vi "Main.vi"(11 "Module Admin":refnum<class "Delacor_lib_QMH_Module Admin.lvclass">) -> ()   [LabVIEW 2023, in "DeviceManager.lvlib"]
doc: "This template is based off of the Queued Message Handler design pattern and the Queued Message Handler project template that ships with LabVIEW.\n\nThe main difference is that the queue is private to this module and communication between modules is performed via Broadcast and Request events.\n\nRequest events are wrapped in public API methods and are handled in the Event Handling Loop (EHL) of this VI. Any module can register for Broadcast events sent by this module. The EHL generates messages based on user interface actions.\n\nThe Message Handling Loop (MHL) processes messages generated by the EHL, or by other messages. The messages are string values, so new messages can be added easily to the Message Cases case structure in the MHL. Each message cluster can also provide an optional value for Message Data, which is a variant that can be converted to whatever message-specific data is required.\n_____\nBased on DQMH Project Template 7.0.0.1280."
uses:
  DeviceManager.lvlib
  <vilib>/Delacor/Delacor QMH/Libraries/Module Admin_class/Delacor_lib_QMH_Module Admin.lvclass
  Module Data--cluster.ctl
  ICLcommuncationData.ctl
  Communicator/Communicator.lvclass
  OpenWebSocketCommunication (Reply Payload)--cluster.ctl
  SendJSONandAskForReply (Reply Payload)--cluster.ctl
  DiscoverDevices (Reply Payload)--cluster.ctl
  Mono/Monochromator.lvclass
  CCD/CCD.lvclass
  SCD/SCD.lvclass
  DevicesList (Reply Payload)--cluster.ctl
  <vilib>/Delacor/Delacor QMH/Libraries/Message Queue_class/Delacor_lib_QMH_Message Queue.lvclass/Delacor_lib_QMH_Message Queue.ctl
  Stop Argument--cluster.ctl
  <vilib>/Delacor/Delacor QMH/Libraries/Module Admin_class/Delacor_lib_QMH_Module Admin.lvclass/Delacor_lib_QMH_Module Admin.ctl
  <vilib>/Utility/miscctls.llb/LVPointTypeDef.ctl
  18cac8b0-4f25-4128-b3b0-f125cc614320.vi
  <vilib>/Delacor/Delacor QMH/Libraries/Message Queue_class/Delacor_lib_QMH_Enqueue Message (Single).vi
  <vilib>/Delacor/Delacor QMH/Libraries/Module Admin_class/Delacor_lib_QMH_Get External Launch.vi
  522d4d4e-e2b9-4a0b-813b-57f0bcdbaa64.vi
  <vilib>/GPower/Error/Library/ErrorType.vi
  <vilib>/GPower/Error/Library/SplitAppended.vi
  <vilib>/Utility/error.llb/Trim Whitespace.vi
  <vilib>/GPower/Error/Library/SubVIs/ExplanationToError.vi
  <vilib>/Utility/error.llb/Trim Whitespace One-Sided.vi
  <vilib>/dlg_ctls.llb/Space Constant.vi
  <vilib>/Utility/error.llb/Error Code Database.vi
  <vilib>/GPower/Error/Library/SubVIs/SetStatus.vi
  <vilib>/GPower/Error/Library/AppendErrors.vi
  <vilib>/GPower/Error/Library/Append/AppendSingle.vi
  <vilib>/Delacor/Delacor QMH/Libraries/Message Queue_class/Delacor_lib_QMH_Message Queue.lvclass
  <vilib>/JKI/JKI DotNet System Exec/dotnet_system_exec/dotnet_system_exec.lvclass
  <vilib>/GPower/Error/GPError.lvlib
panel:
  out "ICL output":string caption="StdErr"
  out "StdOut":string
  out "error out":errorcluster
  out "Status":string
  in  "Simulate MHL Error":bool
  in  "Simulate EHL Error":bool
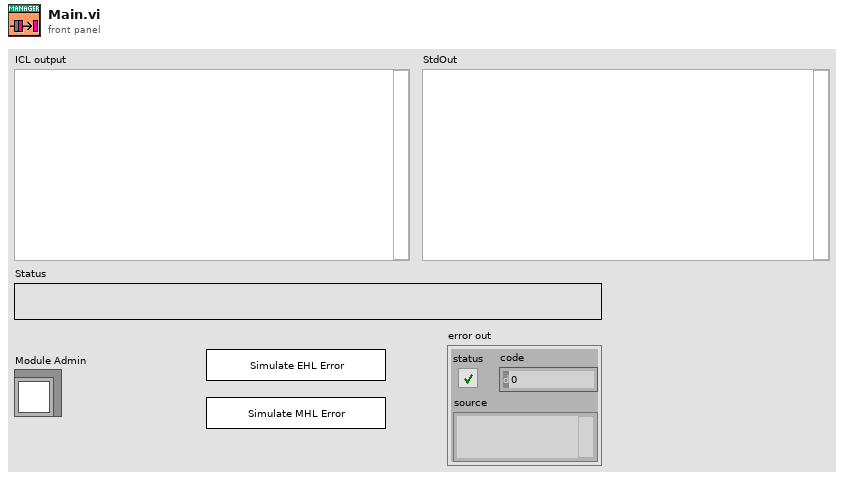
[diagram p1: front panel]
types:
  T1 = cluster{"stdout event":refnum<user-event>, "stderr event":refnum<user-event>, "process_exit event":refnum<user-event>}
  T2 = typedef "DeviceManager.lvlib/Request Events--cluster.ctl" = cluster{"Stop Module":refnum<user-event>, "Show Panel":refnum<user-event>, "Hide Panel":refnum<user-event>, "Get Module Execution Status":refnum<user-event>, "Show Diagram":refnum<user-event>, "StartICL":refnum<user-event>, "OpenWebSocketCommunication":refnum<user-event>, "Private":cluster{"ICLstartNotification":refnum<user-event>}, "ICLshutdown":refnum<user-event>, "SendJSONandAskForReply":refnum<user-event>, "DiscoverDevices":refnum<user-event>, "DevicesList":refnum<user-event>}
  T3 = typedef "DeviceManager.lvlib/ICLcommuncationData.ctl" = cluster{"Status":string, "ICL.exe started":bool, "Communicator":refnum<class "Communicator.lvclass">}
  T4 = typedef "DeviceManager.lvlib/Module Data--cluster.ctl" = cluster{"Status":string}
  T5 = typedef "DeviceManager.lvlib/OpenWebSocketCommunication (Reply Payload)--cluster.ctl" = cluster{"Return Headers":variant, "error":errorcluster}
  T6 = typedef "DeviceManager.lvlib/SendJSONandAskForReply (Reply Payload)--cluster.ctl" = cluster{"JSON reply":string, "error":errorcluster}
  T7 = typedef "DeviceManager.lvlib/DiscoverDevices (Reply Payload)--cluster.ctl" = cluster{"Monos":refnum<class "Monochromator.lvclass">[], "CCDs":refnum<class "CCD.lvclass">[], "SCDs":refnum<class "SCD.lvclass">[], "error":errorcluster}
  T8 = typedef "DeviceManager.lvlib/DevicesList (Reply Payload)--cluster.ctl" = cluster{"monochromator results":string, "CCD-results":string, "SCD-results":string, "error":errorcluster}
  T9 = enum32{"invalid lock state", "Not Locked", "Locked (No Password)", "Password-protected"}
  T10 = typedef "DeviceManager.lvlib/Stop Argument--cluster.ctl" = cluster{"Origin":string, "Exit via Stop Module Req?":bool, "Wait for Module to stop?":bool}
  T11 = typedef "LVPointTypeDef.ctl" = cluster{"Horizontal":i16, "Vertical":i16}
  T12 = enum32{"Invalid", "Standard", "Closed", "Hidden", "Minimized", "Maximized"}
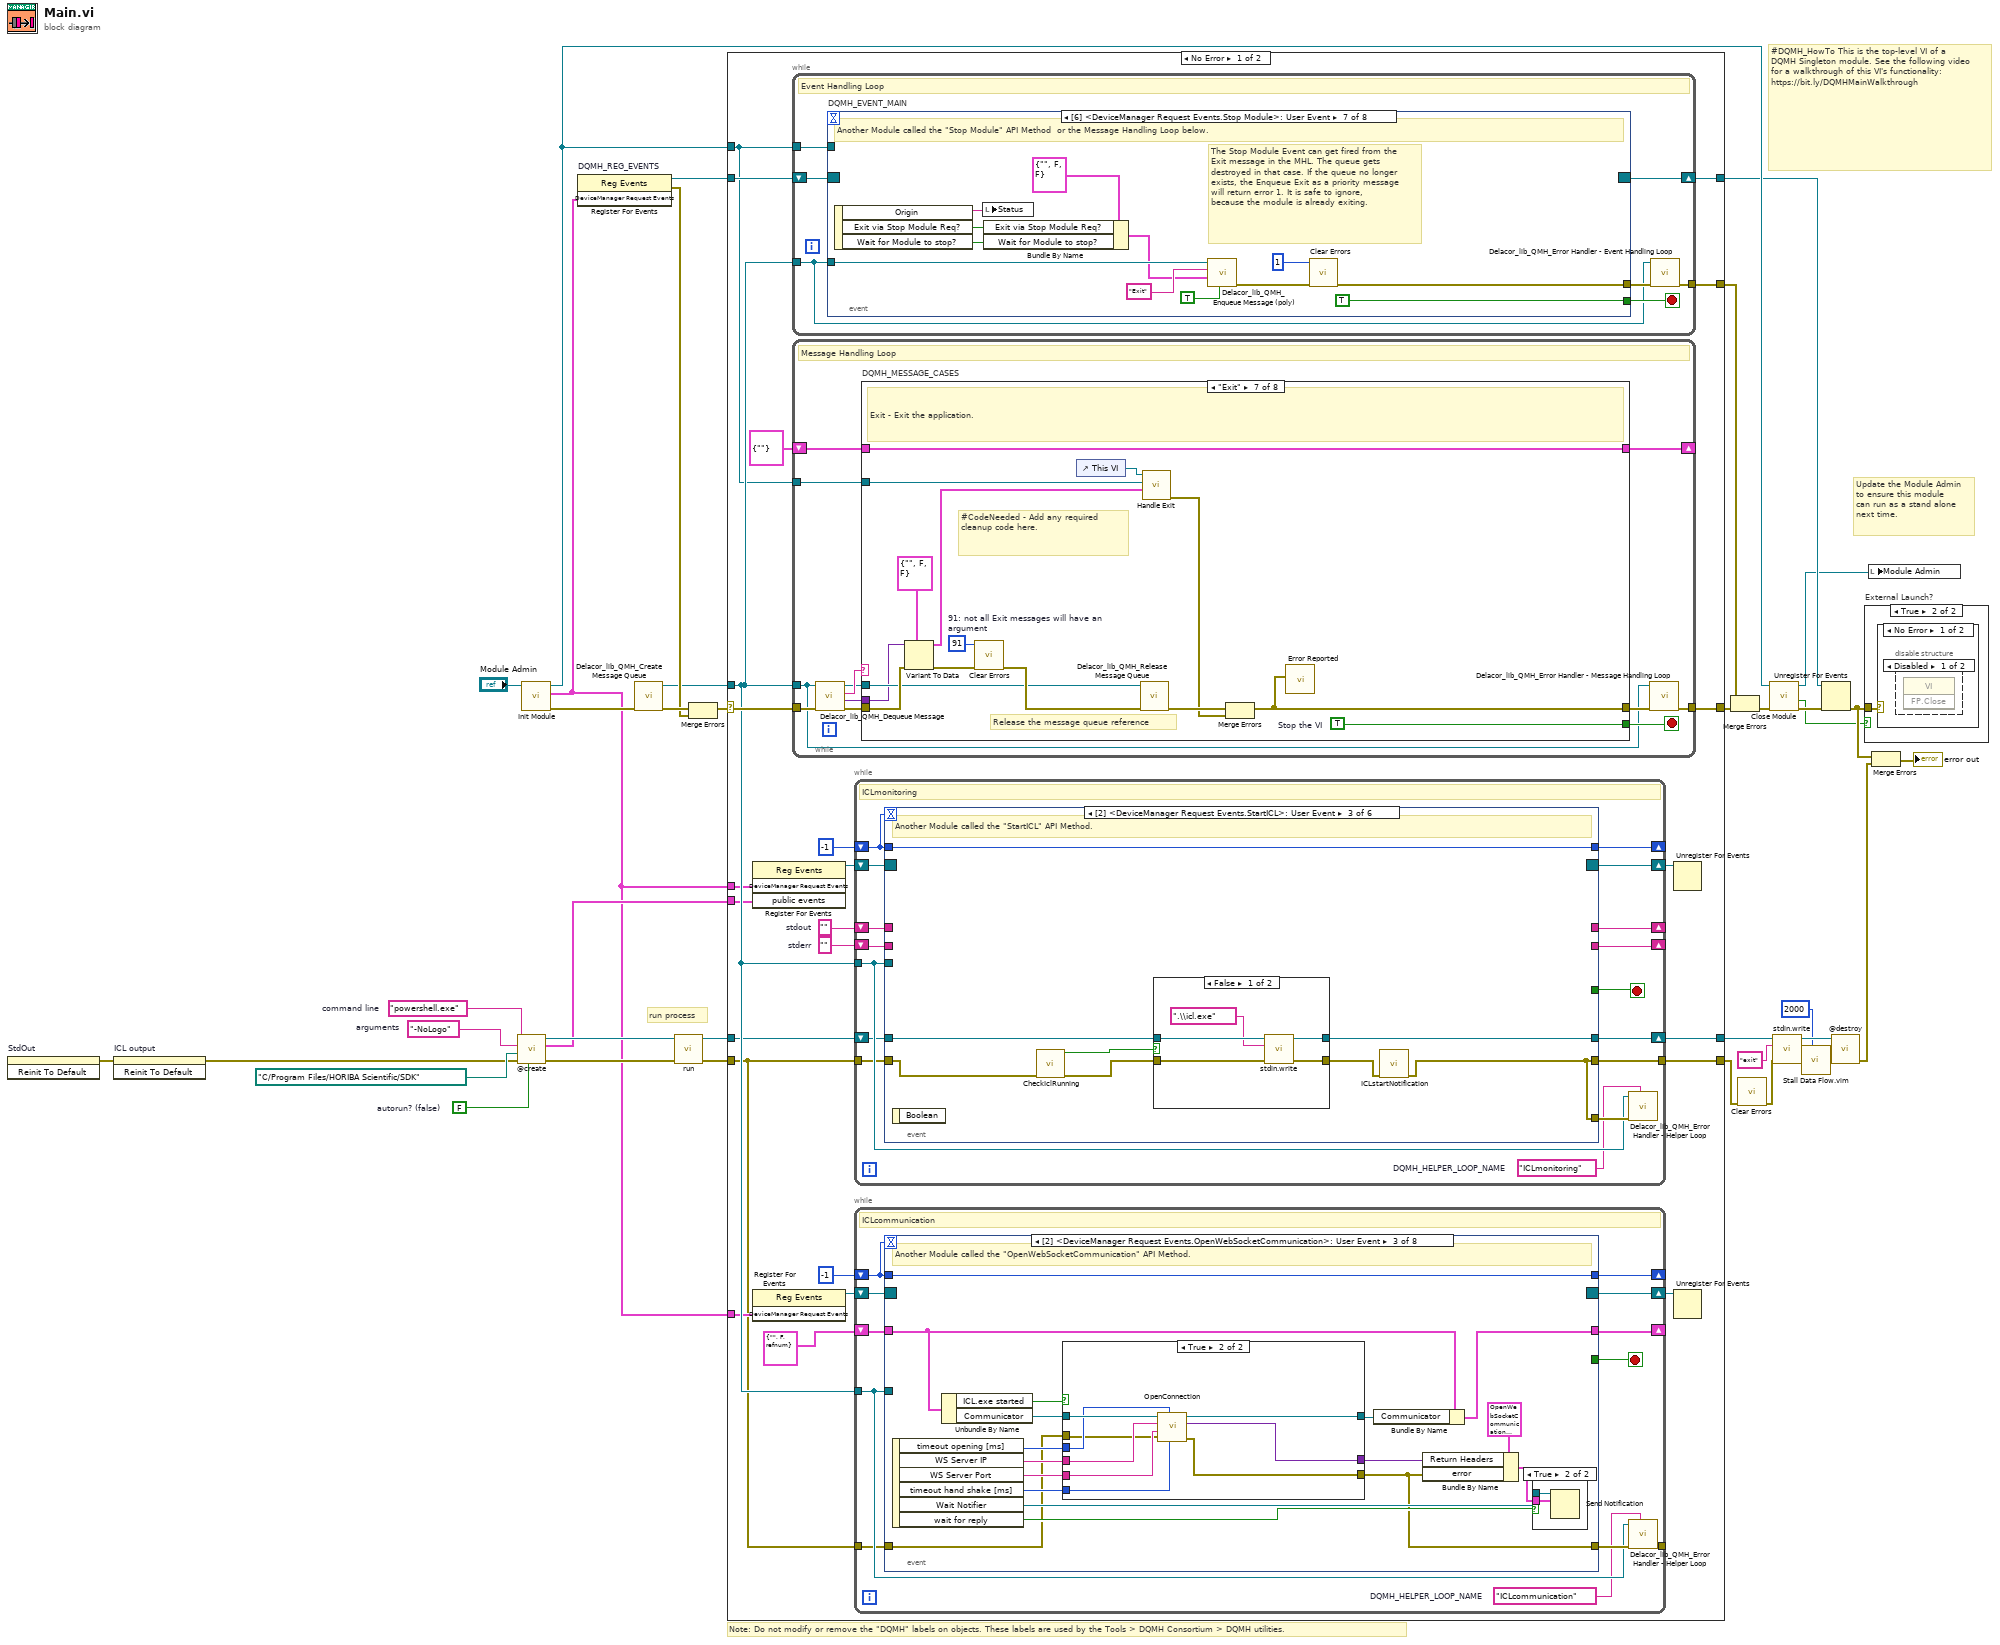
[diagram p0: block diagram]
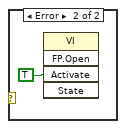
[diagram p4: hidden frame]
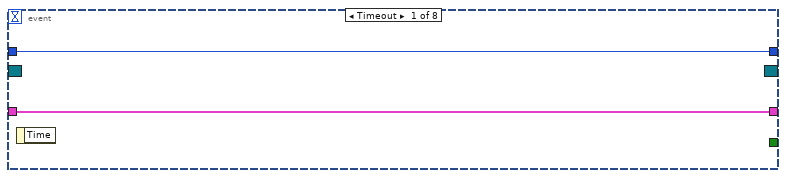
[diagram p5: hidden frame]
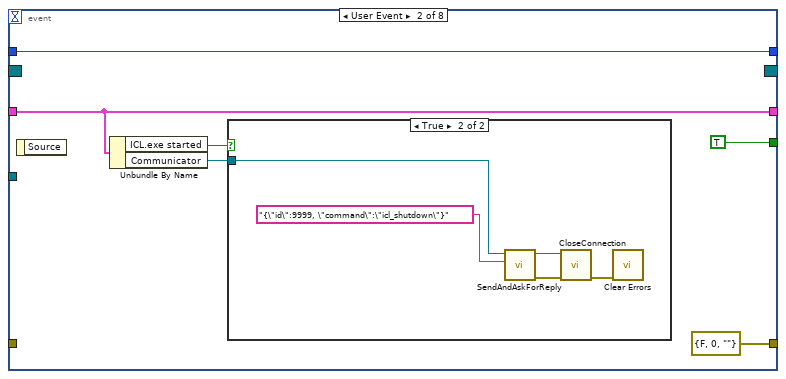
[diagram p6: hidden frame]
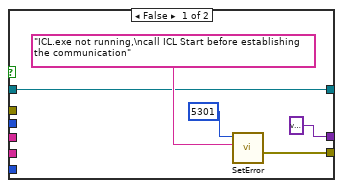
[diagram p8: hidden frame]
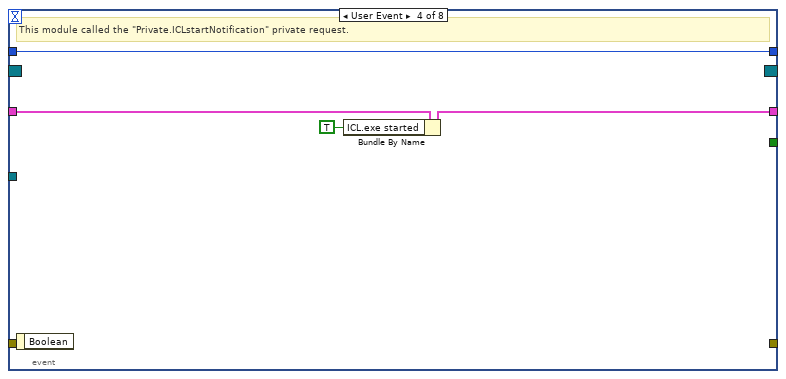
[diagram p10: hidden frame]
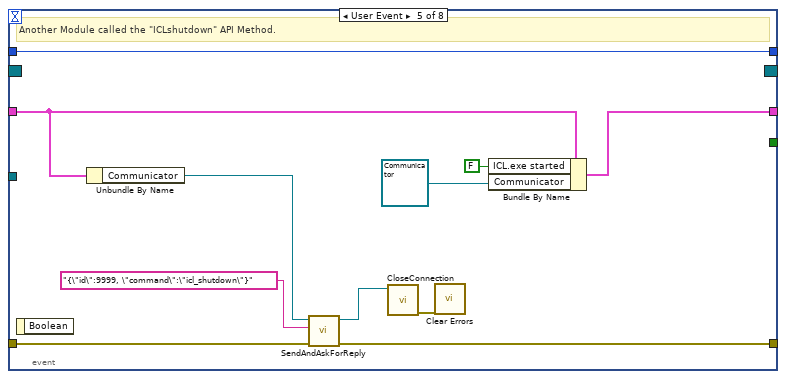
[diagram p11: hidden frame]
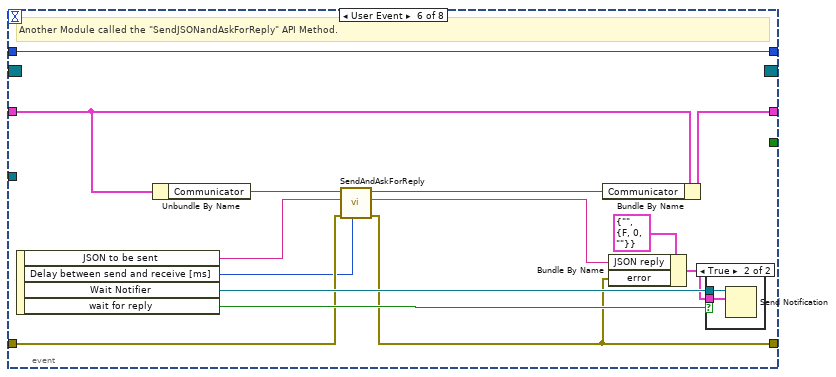
[diagram p12: hidden frame]
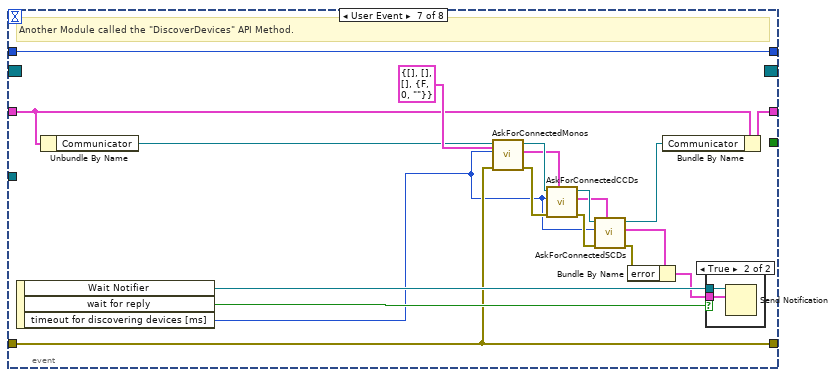
[diagram p14: hidden frame]
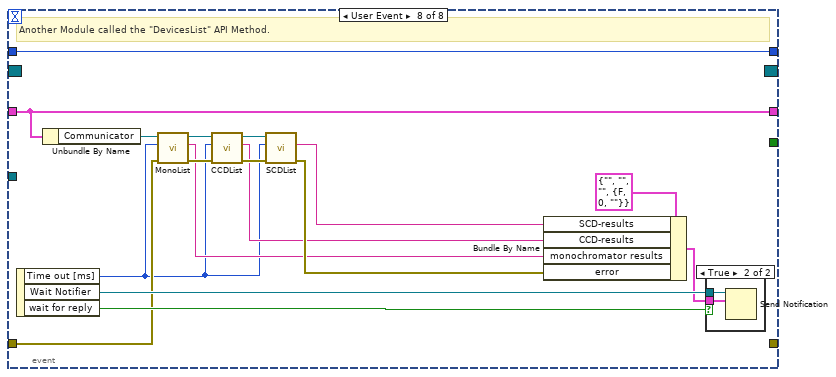
[diagram p16: hidden frame]
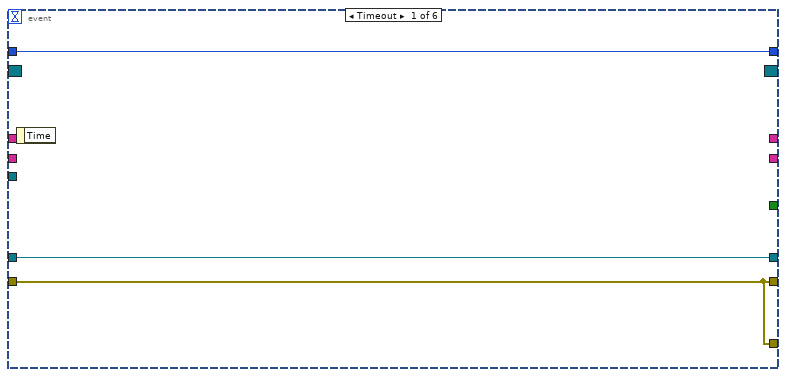
[diagram p18: hidden frame]
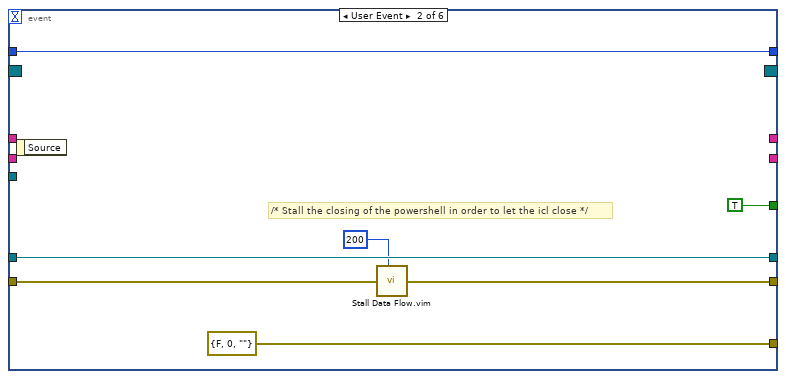
[diagram p19: hidden frame]
diagram:
  w21 = FALSE  # autorun? (false)
  w19 = "-NoLogo"  # arguments
  w18 = "powershell.exe"  # command line
  # "run process"
  # "#DQMH_HowTo This is the top-level VI of a DQMH Singleton module. See the following video for a walkthrough of this VI's functionality: https://bit.ly/DQMHMainWalkthrough"
  # "Note: Do not modify or remove the \"DQMH\" labels on objects. These labels are used by the Tools > DQMH Consortium > DQMH utilities."
  # "Update the Module Admin to ensure this module can run as a stand alone next time."
  n1 = invoke on="StdOut" class="Str" method="Reinit To Default"() -> (error out=w4:errorcluster)  [unwired: 3 in, 2 out]
  n2 = invoke on="ICL output" class="Str" method="Reinit To Default"(error in=w4) -> (error out=w5:errorcluster)  [unwired: 2 in, 2 out]
  n3 = call <vilib>:"@create.vi"("autorun? (false)"=w21, "error in (no error)"=w5, "working directory (c:\\)"=path "C:/Program Files/HORIBA Scientific/SDK" ("working directory"), "arguments (\"\")"=w19, "command line (cmd.exe)"=w18) -> ("error out"=w17:errorcluster, "public events"=w16:T1, "dotnet_system_exec out"=w22:refnum<class "dotnet_system_exec.lvclass">)  [unwired: 4 in]
  n4 = call "Init Module.vi"("Singleton Module Admin in"="Module Admin") -> ("error out"=w37:errorcluster, "DeviceManager Request Events"=w3:T2, "Singleton Module Admin out"=w29:refnum<class "Delacor_lib_QMH_Module Admin.lvclass">)  [unwired: 8 in]
  n5 = register-events "DQMH_REG_EVENTS"(w3) -> (reference out=w27:refnum<event-registration>, error out=w30:errorcluster)  [unwired: 2 in]
  n6 = call <vilib>:"Delacor_lib_QMH_Create Message Queue.vi"("error in"=w37) -> ("error out"=w32:errorcluster, "Message Queue"=w26:refnum<class "Delacor_lib_QMH_Message Queue.lvclass">)  [unwired: 9 in]
  n7 = call <vilib>:"run.vi"("error in (no error)"=w17, "dotnet_system_exec in"=w22) -> ("error out"=w15:errorcluster, "dotnet_system_exec out"=w14:refnum<class "dotnet_system_exec.lvclass">)  [unwired: 8 in]
  n8 = Merge Errors(w32, w30) -> (w31:errorcluster)
  n9 = case shown="No Error" w31 {
    selector: w31 -> [w60 w410]
    tunnel: [w62 w409] -> w38
    tunnel: [w59 w408] -> w28
    tunnel: w27 -> [w57 w408]
    tunnel: w26 -> [w56 w403]
    tunnel: [w61 _] -> w35
    tunnel: w29 -> [w55 w404]
    tunnel: w3 -> [w54 _]
    tunnel: w16 -> [w50 _]
    tunnel: w15 -> [w39 w402]
    tunnel: w14 -> [w49 w401]
    tunnel: [w48 w401] -> w12
    tunnel: [w47 w402] -> w11
    tunnel: w3 -> [w44 _]
    frame No Error {
      w45 = ""  # stderr
      w46 = ""  # stdout
      n10 = register-events ("DQMH_HELPER_REGFOREVENTS")(w54, w50) -> (reference out=w52:refnum<event-registration>)  [unwired: 2 in, 1 out]
      n11 = register-events ("DQMH_HELPER_REGFOREVENTS")(w44) -> (reference out=w42:refnum<event-registration>)  [unwired: 2 in, 1 out]
      n12 = while {
        tunnel: w56 -> [w256]
        shift-right: [w259] -> w59
        shift-left: w57 -> [w260]
        tunnel: [w261] -> w61
        tunnel: w55 -> [w257]
        stop <- w258 stop-if-true
        # "Event Handling Loop"
        n13 = event "DQMH_EVENT_MAIN" shown="[6] <DeviceManager Request Events.Stop Module>: User Event" {
          selector: w260 -> [_ _ _ _ _ _ _ _]
          dyn-events: [_ _ _ _ _ _ _ _] -> w259
          timeout: _ -> [_ _ _ _ _ _ _ _]
          tunnel: [_ _ _ _ _ _ TRUE ("Discard?") _] -> w258
          tunnel: w256 -> [_ w270 _ _ _ _ w294 w301]
          tunnel: [w268 w271 _ _ w277 _ w297 w303] -> w262
          tunnel: w257 -> [_ _ _ _ _ _ _ w300]
          event "Simulate EHL Error": Value Change {
            # "#DQMH_HowTo The 'Simulate EHL Error' button  illustrates how the EHL handles errors. This event is instructional in nature and can be removed."
            # "This case simulates an error being generated by the EHL"
            n14 = event-data() -> ()  [unwired: 1 in, 1 out]
            n15 = call "Module Name--constant.vi"() -> ("Module Name"=w265:string)  [unwired: 11 in]
            n16 = Format Into String(format string="Simulated error originating at Event Handling Loop in %s", w265) -> (resulting string=w266:string)  [unwired: 2 in, 1 out]
            n17 = call <vilib>:"Error Cluster From Error Code.vi"("show call chain? (False)"=TRUE, "error message (\"\")"=w266, "error code (0)"=5000) -> ("error out"=w268:errorcluster)  [unwired: 6 in]
          }
          event "Simulate MHL Error": Value Change {
            # "#DQMH_HowTo The 'Simulate MHL Error' button  illustrates how the MHL handles errors. This event is instructional in nature and can be removed."
            # "This case simulates an error being generated by the MHL"
            n18 = event-data() -> ()  [unwired: 1 in, 1 out]
            n19 = call-poly <vilib>:"Delacor_lib_QMH_Enqueue Message (poly).vi"("Message"="Simulate MHL Error", "Message Queue in"=w270) -> ("error out"=w271:errorcluster)  [unwired: 8 in, 1 out]
          }
          event User Event {
            # "Show the panel of this VI, and send a status updated message to let listeners know."
            # "Another Module called the \"Show Panel\" API Method."
            n20 = event-data() -> ()  [unwired: 1 in, 1 out]
            n21 = control-ref of="This VI"() -> (w273:refnum<vi>)
            n22 = call "Open VI Panel.vi"("VI"=w273) -> ()  [unwired: 10 in, 1 out]
            n23 = call "Status Updated.vi"("Status"="Panel shown." ("format string")) -> ()  [unwired: 10 in, 1 out]
          }
          event User Event {
            # "Hide the panel of this VI, and send a status updated message to let listeners know."
            # "Another Module called the \"Hide Panel\" API Method."
            n24 = event-data() -> ()  [unwired: 1 in, 1 out]
            n25 = control-ref of="This VI"() -> (w275:refnum<vi>)
            n26 = call "Hide VI Panel.vi"("VI"=w275) -> ()  [unwired: 10 in, 1 out]
            n27 = call "Status Updated.vi"("Status"="Panel hidden." ("format string")) -> ()  [unwired: 10 in, 1 out]
          }
          event User Event {
            # "Another Module called the \"Get Module Execution Status\" API Method."
            n28 = event-data() -> ()  [unwired: 1 in, 1 out]
            n29 = call "Update Module Execution Status.vi"("Running?"=TRUE) -> ("error out"=w277:errorcluster)  [unwired: 10 in]
          }
          event User Event {
            # "Another Module called the \"Show Diagram\" API Method. This event is used for debugging."
            n30 = event-data() -> ()  [unwired: 1 in, 1 out]
            n31 = disable-structure shown="RUN_TIME_ENGINE==False" {
              frame condition #0 (active) {
                # "functionality not available in exe"
                n32 = invoke class="VI" method="Lock State.Get"() -> (error out=w283:errorcluster, "Get Lock State"=w282:T9, "pwd in cache"=w279:bool)  [unwired: 4 in, 1 out]
                n33 = Equal?(x=T9."Password-protected", y=w282) -> (x = y?=w280:bool)
                n34 = Compound Arithmetic op=AND(w280, invert w279) -> (w278:bool)
                n35 = case shown="False" w278 {
                  tunnel: w283 -> [w286 _]
                  frame False {
                    n36 = property class="VI"(error in=w286, "BDWin.Open"=TRUE ("Block Diagram Window:Open")) -> ()  [unwired: 1 in, 2 out]
                    n37 = call "Status Updated.vi"("Status"="Block Diagram shown." ("format string")) -> ()  [unwired: 10 in, 1 out]
                  }
                  frame True {
                    # "Password-protected VI, and the password is not in the cache. Do not show the diagram."
                  }
                }
              }
              frame condition #1 {
              }
            }
          }
          event User Event {
            # "The Stop Module Event can get fired from the Exit message in the MHL. The queue gets destroyed in that case. If the queue no longer exists, the Enqueue Exit as a priority message will return error 1. It is safe to ignore, because the module is already exiting."
            # "Another Module called the \"Stop Module\" API Method  or the Message Handling Loop below."
            n38 = event-data() -> ("Origin"=w293:string, "Exit via Stop Module Req?"=w289:bool, "Wait for Module to stop?"=w288:bool)  [unwired: 1 in]
            n39 = local write "Status"(w293) -> ()
            n40 = Bundle By Name(cluster=T10 {"Origin"="", "Exit via Stop Module Req?"=FALSE, "Wait for Module to stop?"=FALSE} ("Stop Argument"), "Exit via Stop Module Req?"=w289, "Wait for Module to stop?"=w288) -> (w287:T10)
            n41 = call-poly <vilib>:"Delacor_lib_QMH_Enqueue Message (poly).vi"("Priority Message? (F)"=TRUE, "Message Data"=w287, "Message"="Exit", "Message Queue in"=w294) -> ("error out"=w298:errorcluster)  [unwired: 6 in, 1 out]
            n42 = call <vilib>:"Clear Errors.vi"("error in (no error)"=w298, "specific error code to clear (0: all)"=1) -> ("error out"=w297:errorcluster)  [unwired: 4 in, 1 out]
          }
          event Panel Close? {
            w302 = TRUE  # Discard the event, the MHL is responsible for closing and stopping this VI.
            # "Hide the panel or send the 'Exit' message if the user clicks the 'X' on the module main VI panel."
            n43 = event-data() -> ()  [unwired: 1 in, 1 out]
            n44 = property class="Module Admin"(reference=w300) -> ("Accessors:External Launch"=w299:bool)  [unwired: 1 in, 2 out]
            n45 = case shown="True" w299 {
              tunnel: w301 -> [_ w309]
              tunnel: [_ w310] -> w303
              frame True {
                # "If externally launched, clicking the 'X' hides the panel, but doesn't close it."
                n46 = control-ref of="This VI"() -> (w306:refnum<vi>)
                n47 = call "Hide VI Panel.vi"("VI"=w306) -> ("error out"=w304:errorcluster)  [unwired: 10 in]
                n48 = call "Status Updated.vi"("error in"=w304, "Status"="Panel hidden." ("format string")) -> ()  [unwired: 9 in, 1 out]
              }
              frame False {
                # "If run as a stand-alone VI, clicking the panel 'X' stops the VI."
                n49 = call-poly <vilib>:"Delacor_lib_QMH_Enqueue Message (poly).vi"("Priority Message? (F)"=TRUE, "Message"="Exit", "Message Queue in"=w309) -> ("error out"=w310:errorcluster)  [unwired: 7 in, 1 out]
              }
            }
            n50 = event-data("Discard?"=w302) -> ()  [unwired: 1 in, 1 out]
          }
        }
        n51 = call-dynamic "Delacor_lib_QMH_Error Handler - Event Handling Loop.vi"("error in"=w262, "Message Queue in"=w256) -> ("dup error in"=w261:errorcluster)  [unwired: 8 in, 1 out]
      }
      n52 = while {
        tunnel: w56 -> [w311]
        shift-right: [w317] -> _
        shift-left: T4 {"Status"=""} ("Data Cluster") -> [w318]
        tunnel: w60 -> [w321]
        tunnel: [w319] -> w62
        tunnel: w55 -> [w312]
        stop <- w316 stop-if-true
        # "Message Handling Loop"
        n53 = call-dynamic "Delacor_lib_QMH_Dequeue Message.vi"("error in"=w321, "Message Queue in"=w311) -> ("error out"=w320:errorcluster, "Message Data"=w314:variant, "Message"=w315:string, "Message Queue out"=w313:refnum<class "Delacor_lib_QMH_Message Queue.lvclass">)  [unwired: 6 in]
        n54 = case "DQMH_MESSAGE_CASES" shown="\"Exit\"" w315 {
          selector: w315 -> [_ _ _ _ _ _ _ w396]
          tunnel: w313 -> [_ _ _ _ _ w362 w384 _]
          tunnel: w320 -> [w340 w344 w347 w349 w358 w369 w390 w399]
          tunnel: [w338 w344 w346 w349 w357 w365 w385 w400] -> w322
          tunnel: w318 -> [w329 w343 w345 w348 w355 w364 w383 w397]
          tunnel: [w328 w343 w345 w348 w355 w364 w383 w397] -> w317
          tunnel: [_ _ _ _ _ _ w382 _] -> w316
          tunnel: w314 -> [_ _ _ _ _ w363 w381 _]
          tunnel: w312 -> [w330 _ _ _ _ w361 w376 _]
          frame "Initialize" {
            w324 = "Initial Message" ("Initial Message")
            # "#CodeNeeded - Initialize the appearance of the front panel."
            # "#CodeNeeded - Initialize your state data here."
            # "Initialize - Any operation that needs to be done before the module can receive messages. Synchronize Caller Events.vi will inform Start Module.vi that the module has launched and is ready to receive messages. Module Did Init.vi will broadcast that the module initialized."
            n55 = call "Synchronize Caller Events.vi"("error in"=w340, "Singleton Module Admin in"=w330) -> ("error out"=w339:errorcluster, "Singleton Module Admin out"=w325:refnum<class "Delacor_lib_QMH_Module Admin.lvclass">)  [unwired: 8 in]
            n56 = property class="Module Admin"(reference=w325) -> ("Accessors:External Launch"=w334:bool)  [unwired: 1 in, 2 out]
            n57 = Select(t=T12."Hidden" ("State"), s=w334, f=T12."Standard" ("State")) -> (s? t:f=w331:T12)
            n58 = call "Module Name--constant.vi"() -> ("Module Name"=w337:string)  [unwired: 11 in]
            n59 = property class="VI"("Front Panel.Title"=w337) -> (reference out=w336:refnum<vi>, error out=w342:errorcluster)  [unwired: 2 in]
            n60 = call "Module Name--constant.vi"() -> ("Module Name"=w326:string)  [unwired: 11 in]
            n61 = invoke class="VI" method="FP.Open"(reference=w336, error in=w342, "State"=w331) -> (reference out=w335:refnum<vi>, error out=w341:errorcluster)  [unwired: 2 in, 3 out]
            n62 = Bundle By Name(cluster=w329, "Status"=w324) -> (w328:T4)
            n63 = call "Module Did Init.vi"("error in"=w339, "Initialized?"=TRUE, "Origin"=w326) -> ("error out"=w338:errorcluster)  [unwired: 8 in]
            n64 = invoke class="VI" method="FP.Center"(reference=w335, error in=w341) -> ()  [unwired: 1 in, 3 out]
            n65 = property on="Pane" class="Pane"("Origin"=T11 {"Horizontal"=0, "Vertical"=0}) -> ()  [unwired: 2 in, 2 out]
            "Status" <- w324
          }
          frame "---Module Specific---" {
            # "Separator -- The following cases handle messages specific to this Module."
          }
          frame "---Copy This Frame---" {
            # "Duplicate this frame when creating new messages.  Change this comment in the duplicated frame to describe this message."
            n66 = Merge Errors(w347) -> (w346:errorcluster)
          }
          frame "---Exit and Error Handling---" {
            # "Separator - The following cases handle errors and exit messages."
          }
          frame "Simulate MHL Error" {
            # "#DQMH_HowTo The 'Simulate MHL Error' button  illustrates how the MHL handles errors. This event is instructional in nature and can be removed."
            # "Simulate an error occurring at the MHL"
            n67 = call "Module Name--constant.vi"() -> ("Module Name"=w351:string)  [unwired: 11 in]
            n68 = Format Into String(format string="Simulated error originating at Message Handling Loop in %s", w351) -> (resulting string=w352:string)  [unwired: 2 in, 1 out]
            n69 = call <vilib>:"Error Cluster From Error Code.vi"("show call chain? (False)"=TRUE, "error message (\"\")"=w352, "error code (0)"=5001) -> ("error out"=w356:errorcluster)  [unwired: 6 in]
            n70 = Merge Errors(w358, w356) -> (w357:errorcluster)
          }
          frame "Error" {
            # "#CodeRecommended - If the module is running in standalone mode (External Launch = FALSE), this code will pop up an error dialog and call the 'Exit' message if an error occurs. Add more fine-grained error management here."
            # "Error - Check the error message data and respond accordingly. This message is sent by the \"Error Handler\" VIs at the end of each loop in this application."
            n71 = property class="Module Admin"(reference=w361) -> ("Accessors:External Launch"=w360:bool)  [unwired: 1 in, 2 out]
            n72 = Variant To Data(error in=w369, type=errorcluster {"status"=FALSE, "code"=0, "source"=""} ("error constant"), Variant=w363) -> (data=w359:errorcluster, error out=w367:errorcluster)
            n73 = local write "error out"(w359) -> ()
            n74 = call "Error Reported.vi"("Error"=w359) -> ()  [unwired: 10 in, 1 out]
            n75 = case shown="False" w360 {
              tunnel: [w374 _] -> w366
              tunnel: w362 -> [w372 _]
              tunnel: w359 -> [w373 _]
              frame False {
                n76 = disable-structure shown="Default" {
                  disable-tunnel: w373 -> [w375 _]
                  frame condition #0 (active) {
                    # "If the module is running standalone, then pop up an error dialog and call the \"Exit\" message."
                    n77 = call <vilib>:"Simple Error Handler.vi"("error in (no error)"=w375) -> ()  [unwired: 4 in, 5 out]
                  }
                  frame condition #1 {
                    # "To prevent the Simple Error Handler VI from being loaded (e.g. when deploying to a Real-Time target), add the Conditional Disable Symbol \"DQMH_Disable_SEH\" to your project and set it to TRUE."
                  }
                }
                n78 = call-poly <vilib>:"Delacor_lib_QMH_Enqueue Message (poly).vi"("Priority Message? (F)"=TRUE, "Message"="Exit", "Message Queue in"=w372) -> ("error out"=w374:errorcluster)  [unwired: 7 in, 1 out]
              }
              frame True {
                # "If the module was launched externally, calling the Error Reported broadcast VI is the only action performed by the \"Error\" message. The module's caller can then process the error appropriately."
              }
            }
            n79 = Merge Errors(w367, w366) -> (w365:errorcluster)
          }
          frame "Exit" {
            w380 = 91  # 91: not all Exit messages will have an argument
            w382 = TRUE  # Stop the VI
            # "Release the message queue reference"
            # "#CodeNeeded - Add any required cleanup code here."
            # "Exit - Exit the application."
            n80 = Variant To Data(error in=w390, type=T10 {"Origin"="", "Exit via Stop Module Req?"=FALSE, "Wait for Module to stop?"=FALSE} ("Stop Argument"), Variant=w381) -> (data=w378:T10, error out=w387:errorcluster)
            n81 = call <vilib>:"Clear Errors.vi"("error in (no error)"=w387, "specific error code to clear (0: all)"=w380) -> ("error out"=w389:errorcluster)  [unwired: 4 in, 1 out]
            n82 = control-ref of="This VI"() -> (w377:refnum<vi>)
            n83 = call-dynamic "Delacor_lib_QMH_Release Message Queue.vi"("error in"=w389, "Message Queue"=w384) -> ("error out"=w388:errorcluster)  [unwired: 9 in]
            n84 = call "Handle Exit.vi"("Stop Argument"=w378, "Admin in"=w376, "VI reference"=w377) -> ("error out"=w386:errorcluster)  [unwired: 7 in, 1 out]
            n85 = Merge Errors(w388, w386) -> (w385:errorcluster)
            n86 = call "Error Reported.vi"("Error"=w385) -> ()  [unwired: 10 in, 1 out]
          }
          frame Default {
            # "'Default' case only runs if there is a message that isn't defined in any of the other cases.  Output a programming error."
            n87 = call "Module Name--constant.vi"() -> ("Module Name"=w395:string)  [unwired: 11 in]
            n88 = Format Into String(format string="The invalid message string \"%s\" was received in the Message Handling Loop for module \"%s\".", w396, w395) -> (resulting string=w391:string)  [unwired: 2 in, 1 out]
            n89 = call <vilib>:"Error Cluster From Error Code.vi"("show call chain? (False)"=TRUE, "error message (\"\")"=w391, "error code (0)"=1) -> ("error out"=w398:errorcluster)  [unwired: 6 in]
            n90 = Merge Errors(w399, w398) -> (w400:errorcluster)
          }
        }
        n91 = call-dynamic "Delacor_lib_QMH_Error Handler - Message Handling Loop.vi"("error in"=w322, "Message Queue in"=w311) -> ("dup error in"=w319:errorcluster)  [unwired: 8 in, 1 out]
      }
      n92 = while "DQMH_HELPER_LOOP" {
        shift-right: [w207] -> _
        shift-left: -1 -> [w206]
        shift-right: [w204] -> w53
        shift-left: w52 -> [w205]
        tunnel: w56 -> [w201]
        tunnel: w39 -> [w199]
        shift-right: [w196] -> w48
        shift-left: w49 -> [w198]
        tunnel: [w197] -> w47
        shift-right: [w192] -> _
        shift-left: w46 -> [w193]
        shift-right: [w195] -> _
        shift-left: w45 -> [w194]
        stop <- w203 stop-if-true
        w200 = "ICLmonitoring"  # DQMH_HELPER_LOOP_NAME
        # "ICLmonitoring"
        n93 = event "DQMH_HELPER_EVENT_STRUCTURE" shown="[2] <DeviceManager Request Events.StartICL>: User Event" {
          selector: w205 -> [_ _ _ _ _ _]
          dyn-events: [_ _ _ _ _ _] -> w204
          timeout: w206 -> [_ _ _ _ _ _]
          tunnel: w206 -> [w210 w217 w225 w241 w251 w255]
          tunnel: [w210 w217 w225 w241 w251 w255] -> w207
          tunnel: [_ TRUE _ _ _ TRUE] -> w203
          tunnel: [w208 errorcluster {"status"=FALSE, "code"=0, "source"=""} ("error constant") w221 _ _ _] -> w202
          tunnel: w201 -> [_ _ _ _ _ _]
          tunnel: w199 -> [w208 w213 w220 _ w242 w252]
          tunnel: w198 -> [w209 w214 w223 w240 w250 w254]
          tunnel: [w208 w212 w221 _ w242 w252] -> w197
          tunnel: [w209 w214 w224 w240 w250 w254] -> w196
          tunnel: [_ _ _ w239 w245 _] -> w195
          tunnel: w194 -> [_ _ _ w239 w248 _]
          tunnel: w193 -> [_ _ _ w237 w246 _]
          tunnel: [_ _ _ w235 w246 _] -> w192
          event Timeout {
            n94 = event-data() -> ()  [unwired: 1 in, 1 out]
          }
          event User Event {
            # "/* Stall the closing of the powershell in order to let the icl close */"
            n95 = event-data() -> ()  [unwired: 1 in, 1 out]
            n96 = call "Stall Data Flow.vim"("value in"=w213, "milliseconds to wait"=u32 200) -> ("value out"=w212:errorcluster)  [unwired: 1 out]
          }
          event User Event {
            # "Another Module called the \"StartICL\" API Method."
            n97 = event-data() -> ()  [unwired: 1 in, 1 out]
            n98 = call "CheckIclRunning.vi"("error in (no error)"=w220) -> ("error out"=w218:errorcluster, "icl.exe running"=w219:bool)  [unwired: 9 in]
            n99 = case shown="False" w219 {
              tunnel: [w230 w232] -> w224
              tunnel: w223 -> [w229 w232]
              tunnel: [w227 w231] -> w222
              tunnel: w218 -> [w226 w231]
              frame False {
                n100 = call-dynamic "stdin.write.vi"("error in (no error)"=w226, "stdin"=".\\icl.exe", "dotnet_system_exec in"=w229) -> ("error out"=w227:errorcluster, "dotnet_system_exec out"=w230:refnum<class "dotnet_system_exec.lvclass">)  [unwired: 7 in]
              }
              frame True {
              }
            }
            n101 = call "ICLstartNotification.vi"("error in"=w222) -> ("error out"=w221:errorcluster)  [unwired: 10 in]
          }
          event User Event {
            n102 = event-data() -> ("StdOut Event"=w236:string)  [unwired: 1 in]
            n103 = Concatenate Strings(w237, "\n", w236) -> (w235:string)
            "StdOut" <- w235
            n104 = control-ref of="StdOut"() -> (w234:refnum<vi>)
            n105 = property on="Property Node" class="Str"(reference=w234, "Text.Scroll Position"=u32 4294967295) -> ()  [unwired: 1 in, 2 out]
          }
          event User Event {
            n106 = event-data() -> ("StdErr Event"=w247:string)  [unwired: 1 in]
            n107 = Concatenate Strings(w248, "\n", w247) -> (w245:string)
            "ICL output" <- w245
            n108 = control-ref of="ICL output"() -> (w243:refnum<vi>)
            n109 = property on="Property Node" class="Str"(reference=w243, "Text.Scroll Position"=u32 4294967295) -> ()  [unwired: 1 in, 2 out]
          }
          event User Event {
            n110 = event-data() -> ()  [unwired: 1 in, 1 out]
          }
        }
        n111 = call-dynamic "Delacor_lib_QMH_Error Handler - Helper Loop.vi"("Error Debug"=w200, "error in"=w202, "Message Queue in"=w201) -> ()  [unwired: 7 in, 2 out]
      }
      n112 = while "DQMH_HELPER_LOOP" {
        shift-right: [w74] -> _
        shift-left: -1 -> [w73]
        shift-right: [w71] -> w43
        shift-left: w42 -> [w72]
        tunnel: w56 -> [w68]
        shift-right: [w65] -> _
        shift-left: T3 {"Status"="", "ICL.exe started"=FALSE, "Communicator"=refnum} ("Data Cluster") -> [w66]
        tunnel: [w64] -> _
        tunnel: w39 -> [w63]
        stop <- w70 stop-if-true
        w67 = "ICLcommunication"  # DQMH_HELPER_LOOP_NAME
        # "ICLcommunication"
        n113 = event "DQMH_HELPER_EVENT_STRUCTURE" shown="[2] <DeviceManager Request Events.OpenWebSocketCommunication>: User Event" {
          selector: w72 -> [_ _ _ _ _ _ _ _]
          dyn-events: [_ _ _ _ _ _ _ _] -> w71
          timeout: w73 -> [_ _ _ _ _ _ _ _]
          tunnel: w73 -> [w76 w82 w104 w124 w135 w149 w170 w189]
          tunnel: [w76 w82 w104 w124 w135 w149 w170 w189] -> w74
          tunnel: [_ TRUE _ _ _ _ _ _] -> w70
          tunnel: [_ errorcluster {"status"=FALSE, "code"=0, "source"=""} ("error constant") w89 _ w125 w139 w158 _] -> w69
          tunnel: w68 -> [_ _ _ _ _ _ _ _]
          tunnel: w66 -> [w75 w78 w91 w123 w128 w144 w155 w173]
          tunnel: [w75 w78 w92 w122 w129 w138 w154 w173] -> w65
          tunnel: w63 -> [_ _ w88 _ w132 w141 w158 w183]
          event Timeout {
            n114 = event-data() -> ()  [unwired: 1 in, 1 out]
          }
          event User Event {
            n115 = event-data() -> ()  [unwired: 1 in, 1 out]
            n116 = Unbundle By Name(w78) -> ("ICL.exe started"=w77:bool, "Communicator"=w79:refnum<class "Communicator.lvclass">)
            n117 = case shown="True" w77 {
              tunnel: w79 -> [_ w87]
              frame False {
              }
              frame True {
                n118 = call-dynamic "SendAndAskForReply.vi"("String to be sent"="{\"id\":9999, \"command\":\"icl_shutdown\"}", "Communicator in"=w87) -> ("error out"=w84:errorcluster, "Communicator out"=w85:refnum<class "Communicator.lvclass">)  [unwired: 7 in, 1 out]
                n119 = call-dynamic "CloseConnection.vi"("error in (no error)"=w84, "Communicator in"=w85) -> ("error out"=w83:errorcluster)  [unwired: 8 in, 1 out]
                n120 = call <vilib>:"Clear Errors.vi"("error in (no error)"=w83) -> ()  [unwired: 5 in, 2 out]
              }
            }
          }
          event User Event {
            # "Another Module called the \"OpenWebSocketCommunication\" API Method."
            n121 = event-data() -> ("timeout opening [ms]"=w93:i32, "WS Server IP"=w95:string, "WS Server Port"=w96:string, "timeout hand shake [ms]"=w94:i32, "Wait Notifier"=w103:refnum<notifier>, "wait for reply"=w102:bool)  [unwired: 1 in]
            n122 = Unbundle By Name(w91) -> ("ICL.exe started"=w99:bool, "Communicator"=w97:refnum<class "Communicator.lvclass">)
            n123 = case shown="True" w99 {
              tunnel: [w107 w113] -> w89
              tunnel: [variant ("Return Headers") w112] -> w98
              tunnel: w97 -> [w105 w118]
              tunnel: w96 -> [_ w117]
              tunnel: w95 -> [_ w116]
              tunnel: w94 -> [_ w115]
              tunnel: w93 -> [_ w114]
              tunnel: [w105 w111] -> w90
              tunnel: w88 -> [_ w110]
              frame False {
                n124 = call <vilib>:"SetError.vi"("Error description"="ICL.exe not running,\ncall ICL Start before establishing the communication", "Error code"=5301) -> ("Error out"=w107:errorcluster)  [unwired: 9 in]
              }
              frame True {
                n125 = call-dynamic "OpenConnection.vi"("timeout hand shake [ms]"=w115, "timeout opening [ms]"=w114, "error in (no error)"=w110, "WS Server Port"=w117, "WS Server IP"=w116, "Communicator in"=w118) -> ("error out"=w113:errorcluster, "Return Headers"=w112:variant, "Communicator out"=w111:refnum<class "Communicator.lvclass">)  [unwired: 3 in]
              }
            }
            n126 = Bundle By Name(cluster=w91, "Communicator"=w90) -> (w92:T3)
            n127 = Bundle By Name(cluster=T5 {"Return Headers"=variant, "error"={"status"=FALSE, "code"=0, "source"=""}} ("OpenWebSocketCommunication (Reply Payload)"), "Return Headers"=w98, "error"=w89) -> (w101:T5)
            n128 = case "DQMH_FIRE_NOTIFIER" shown="True" w102 {
              tunnel: w103 -> [_ w120]
              tunnel: w101 -> [_ w119]
              frame False {
              }
              frame True {
                n129 = Send Notification(notification=w119, notifier=w120) -> ()  [unwired: 1 in, 2 out]
              }
            }
          }
          event User Event {
            # "This module called the \"Private.ICLstartNotification\" private request."
            n130 = event-data() -> ()  [unwired: 1 in, 1 out]
            n131 = Bundle By Name(cluster=w123, "ICL.exe started"=TRUE) -> (w122:T3)
          }
          event User Event {
            # "Another Module called the \"ICLshutdown\" API Method."
            n132 = event-data() -> ()  [unwired: 1 in, 1 out]
            n133 = Unbundle By Name(w128) -> ("Communicator"=w134:refnum<class "Communicator.lvclass">)
            n134 = call-dynamic "SendAndAskForReply.vi"("error in (no error)"=w132, "String to be sent"="{\"id\":9999, \"command\":\"icl_shutdown\"}", "Communicator in"=w134) -> ("error out"=w125:errorcluster, "Communicator out"=w131:refnum<class "Communicator.lvclass">)  [unwired: 6 in, 1 out]
            n135 = call-dynamic "CloseConnection.vi"("Communicator in"=w131) -> ("error out"=w130:errorcluster)  [unwired: 9 in, 1 out]
            n136 = call <vilib>:"Clear Errors.vi"("error in (no error)"=w130) -> ()  [unwired: 5 in, 2 out]
            n137 = Bundle By Name(cluster=w128, "ICL.exe started"=FALSE, "Communicator"=refnum<class "Communicator.lvclass"> refnum) -> (w129:T3)
          }
          event User Event {
            # "Another Module called the \"SendJSONandAskForReply\" API Method."
            n138 = event-data() -> ("JSON to be sent"=w142:string, "Delay between send and receive [ms]"=w136:i32, "Wait Notifier"=w148:refnum<notifier>, "wait for reply"=w147:bool)  [unwired: 1 in]
            n139 = Unbundle By Name(w144) -> ("Communicator"=w143:refnum<class "Communicator.lvclass">)
            n140 = call-dynamic "SendAndAskForReply.vi"("Delay between send and receive [ms]"=w136, "error in (no error)"=w141, "String to be sent"=w142, "Communicator in"=w143) -> ("error out"=w139:errorcluster, "Data"=w140:string, "Communicator out"=w137:refnum<class "Communicator.lvclass">)  [unwired: 5 in]
            n141 = Bundle By Name(cluster=w144, "Communicator"=w137) -> (w138:T3)
            n142 = Bundle By Name(cluster=T6 {"JSON reply"="", "error"={"status"=FALSE, "code"=0, "source"=""}} ("SendJSONandAskForReply (Reply Payload)"), "JSON reply"=w140, "error"=w139) -> (w146:T6)
            n143 = case "DQMH_FIRE_NOTIFIER" shown="True" w147 {
              tunnel: w148 -> [_ w151]
              tunnel: w146 -> [_ w150]
              frame False {
              }
              frame True {
                n144 = Send Notification(notification=w150, notifier=w151) -> ()  [unwired: 1 in, 2 out]
              }
            }
          }
          event User Event {
            # "Another Module called the \"DiscoverDevices\" API Method."
            n145 = event-data() -> ("Wait Notifier"=w169:refnum<notifier>, "wait for reply"=w168:bool, "timeout for discovering devices [ms]"=w152:i32)  [unwired: 1 in]
            n146 = Unbundle By Name(w155) -> ("Communicator"=w161:refnum<class "Communicator.lvclass">)
            n147 = call "AskForConnectedMonos.vi"("DiscoverDevices in"=T7 {"Monos"=[], "CCDs"=[], "SCDs"=[], "error"={"status"=FALSE, "code"=0, "source"=""}}, "error in (no error)"=w158, "timeout for receiving data [ms]"=w152, "Communicator in"=w161) -> ("error out"=w157:errorcluster, "DiscoverDevices out"=w159:T7, "Communicator out"=w160:refnum<class "Communicator.lvclass">)  [unwired: 5 in]
            n148 = call "AskForConnectedCCDs.vi"("DiscoverDevices in"=w159, "error in (no error)"=w157, "timeout for receiving data [ms]"=w152, "Communicator in"=w160) -> ("error out"=w165:errorcluster, "DiscoverDevices out"=w166:T7, "Communicator out"=w167:refnum<class "Communicator.lvclass">)  [unwired: 5 in]
            n149 = call "AskForConnectedSCDs.vi"("DiscoverDevices in"=w166, "error in (no error)"=w165, "timeout for receiving data [ms]"=w152, "Communicator in"=w167) -> ("error out"=w164:errorcluster, "DiscoverDevices out"=w163:T7, "Communicator out"=w153:refnum<class "Communicator.lvclass">)  [unwired: 5 in]
            n150 = Bundle By Name(cluster=w163, "error"=w164) -> (w156:T7)
            n151 = Bundle By Name(cluster=w155, "Communicator"=w153) -> (w154:T3)
            n152 = case "DQMH_FIRE_NOTIFIER" shown="True" w168 {
              tunnel: w169 -> [_ w172]
              tunnel: w156 -> [_ w171]
              frame False {
              }
              frame True {
                n153 = Send Notification(notification=w171, notifier=w172) -> ()  [unwired: 1 in, 2 out]
              }
            }
          }
          event User Event {
            # "Another Module called the \"DevicesList\" API Method."
            n154 = event-data() -> ("Time out [ms]"=w174:i32, "Wait Notifier"=w188:refnum<notifier>, "wait for reply"=w187:bool)  [unwired: 1 in]
            n155 = Unbundle By Name(w173) -> ("Communicator"=w184:refnum<class "Communicator.lvclass">)
            n156 = call "MonoList.vi"("error in (no error)"=w183, "Delay between send and receive [ms]"=w174, "Communicator in"=w184) -> ("error out"=w180:errorcluster, "results-JSON"=w175:string, "Communicator out"=w182:refnum<class "Communicator.lvclass">)  [unwired: 5 in, 1 out]
            n157 = call "CCDList.vi"("error in (no error)"=w180, "Delay between send and receive [ms]"=w174, "Communicator in"=w182) -> ("error out"=w179:errorcluster, "results-JSON"=w177:string, "Communicator out"=w181:refnum<class "Communicator.lvclass">)  [unwired: 5 in, 1 out]
            n158 = call "SCDList.vi"("error in (no error)"=w179, "Delay between send and receive [ms]"=w174, "Communicator in"=w181) -> ("error out"=w178:errorcluster, "results-JSON"=w176:string)  [unwired: 5 in, 2 out]
            n159 = Bundle By Name(cluster=T8 {"monochromator results"="", "CCD-results"="", "SCD-results"="", "error"={"status"=FALSE, "code"=0, "source"=""}} ("DevicesList (Reply Payload)"), "SCD-results"=w176, "CCD-results"=w177, "monochromator results"=w175, "error"=w178) -> (w186:T8)
            n160 = case "DQMH_FIRE_NOTIFIER" shown="True" w187 {
              tunnel: w188 -> [_ w191]
              tunnel: w186 -> [_ w190]
              frame False {
              }
              frame True {
                n161 = Send Notification(notification=w190, notifier=w191) -> ()  [unwired: 1 in, 2 out]
              }
            }
          }
        }
        n162 = call-dynamic "Delacor_lib_QMH_Error Handler - Helper Loop.vi"("Error Debug"=w67, "error in"=w69, "Message Queue in"=w68) -> ("dup error in"=w64:errorcluster)  [unwired: 7 in, 1 out]
      }
      n163 = Unregister For Events(event registration refnum=w53) -> ()  [unwired: 1 in, 1 out]
      n164 = Unregister For Events(event registration refnum=w43) -> ()  [unwired: 1 in, 1 out]
    }
    frame Error {
      # "Synchronize Caller Events.vi will inform Start Module.vi that the module has launched and will let the code calling Start Module.vi register for broadcasts and would permit the caller receive the broadcast that an error occurred at launch time."
      n165 = call-dynamic "Delacor_lib_QMH_Release Message Queue.vi"("error in"=w410, "Message Queue"=w403) -> ("error out"=w409:errorcluster)  [unwired: 9 in]
      n166 = call "Synchronize Caller Events.vi"("Singleton Module Admin in"=w404) -> ("error out"=w411:errorcluster)  [unwired: 9 in, 1 out]
      n167 = call "Module Name--constant.vi"() -> ("Module Name"=w407:string)  [unwired: 11 in]
      n168 = Format Into String(format string="An error occurred during initialization. %s is no longer running.", w407) -> (resulting string=w405:string)  [unwired: 2 in, 1 out]
      n169 = Merge Errors(w409, w411) -> (w412:errorcluster)
      n170 = call "Error Reported.vi"("Additional Information"=w405, "Error"=w412) -> ()  [unwired: 9 in, 1 out]
    }
  }
  n171 = Merge Errors(w35, w38) -> (w34:errorcluster)
  n172 = call <vilib>:"Clear Errors.vi"("error in (no error)"=w11) -> ("error out"=w7:errorcluster)  [unwired: 5 in, 1 out]
  n173 = call "Close Module.vi"("error in"=w34, "Module Admin in"=w29) -> ("error out"=w36:errorcluster, "External Launch"=w23:bool, "Module Admin out"=w24:refnum<class "Delacor_lib_QMH_Module Admin.lvclass">)  [unwired: 7 in]
  n174 = call-dynamic "stdin.write.vi"("error in (no error)"=w7, "stdin"="exit", "dotnet_system_exec in"=w12) -> ("error out"=w13:errorcluster, "dotnet_system_exec out"=w10:refnum<class "dotnet_system_exec.lvclass">)  [unwired: 7 in]
  n175 = call "Stall Data Flow.vim"("value in"=w13, "milliseconds to wait"=u32 2000) -> ("value out"=w2:errorcluster)  [unwired: 1 out]
  n176 = Unregister For Events(event registration refnum=w28, error in=w36) -> (error out=w33:errorcluster)
  n177 = call-dynamic "@destroy.vi"("error in (no error)"=w2, "dotnet_system_exec in"=w10) -> ("error out"=w8:errorcluster)  [unwired: 8 in, 1 out]
  n178 = case "External Launch?" shown="True" w23 {
    tunnel: w33 -> [_ w413]
    frame False {
    }
    frame True {
      n179 = case shown="No Error" w413 {
        frame No Error {
          n180 = disable-structure shown="Disabled" {
            frame Disabled {
              n181 = invoke class="VI" method="FP.Close"() -> ()  [unwired: 3 in, 3 out]
            }
            frame Enabled {
            }
          }
        }
        frame Error {
          n182 = invoke class="VI" method="FP.Open"("Activate"=TRUE ("Activate?")) -> ()  [unwired: 4 in, 5 out]
        }
      }
    }
  }
  n183 = local write "Module Admin"(w24) -> ()
  n184 = Merge Errors(w33, w8) -> (→"error out":errorcluster)
